vi "Set AutoClear.vi"(8 "error in (no error)":errorcluster, 10 "AutoClear":bool, 11 "App Settings in":refnum<class "App Settings.lvclass">) -> (0 "error out":errorcluster, 3 "App Settings out":refnum<class "App Settings.lvclass">)   [LabVIEW 2015, in "Application.lvlib" / "App Settings.lvclass"]
uses:
  App Settings.lvclass
  App Settings.lvclass/App Settings.ctl
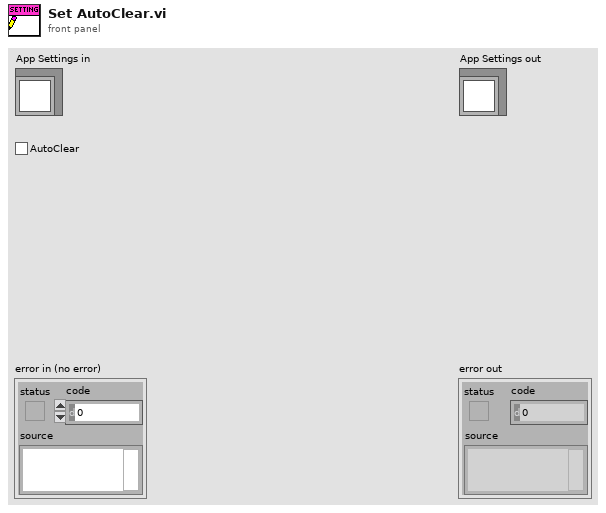
[diagram p1: front panel]
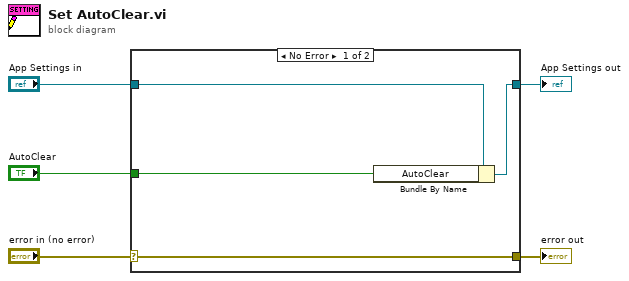
[diagram p0: block diagram]
diagram:
  n1 = case shown="No Error" "error in (no error)" {
    selector: "error in (no error)" -> [w9 w10]
    tunnel: [w9 w10] -> w4
    tunnel: [w7 w11] -> w2
    tunnel: "App Settings in" -> [w8 w11]
    tunnel: "AutoClear" -> [w6 _]
    frame No Error {
      n2 = Bundle By Name(cluster=w8, "AutoClear"=w6) -> (w7:refnum<class "App Settings.lvclass">)
    }
    frame Error {
    }
  }
  "error out" <- w4
  "App Settings out" <- w2
